vi "Read Parent Attributes.vi"(11 "Attributes in":refnum<class "Attributes.lvclass">) -> (2 "Parent Attributes":refnum<class "Attributes.lvclass">)   [LabVIEW 2025, in "jettl.lvlib" / "Attributes.lvlib" / "Attributes.lvclass"]
uses:
  Attributes.lvclass
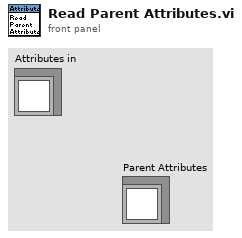
[diagram p1: front panel]
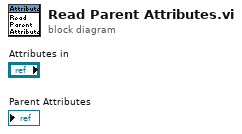
[diagram p0: block diagram]
diagram:
